vi "HW_Poll_Tracker.vi"(0 "VISA resource name in":refnum<visa-resource-name>="ASRL3::INSTR", 11 "error in":errorcluster) -> (1 "Binary mode status":string, 2 "Coordinate mode status":string, 3 "Matrix mode status":string, 4 "VISA resource name out":refnum<visa-resource-name>, 10 "Read buffer":string, 12 "Sensors response":string, 13 "FPS status":i32, 14 "Port data status":i32, 15 "error out":errorcluster)   [LabVIEW 2016]
panel:
  out "Port data status index":i32
  out "Poll records":u32
  out "FPS target index":i32
  out "Matrix mode index":i32
  out "Coordinate mode index":i32
  out "Binary mode index":i32
  out "Array of tokens":string[](array[string])
  out "token index":i32
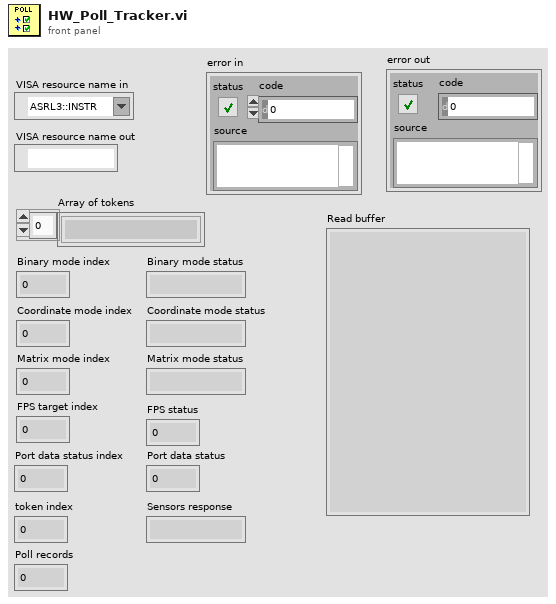
[diagram p1: front panel]
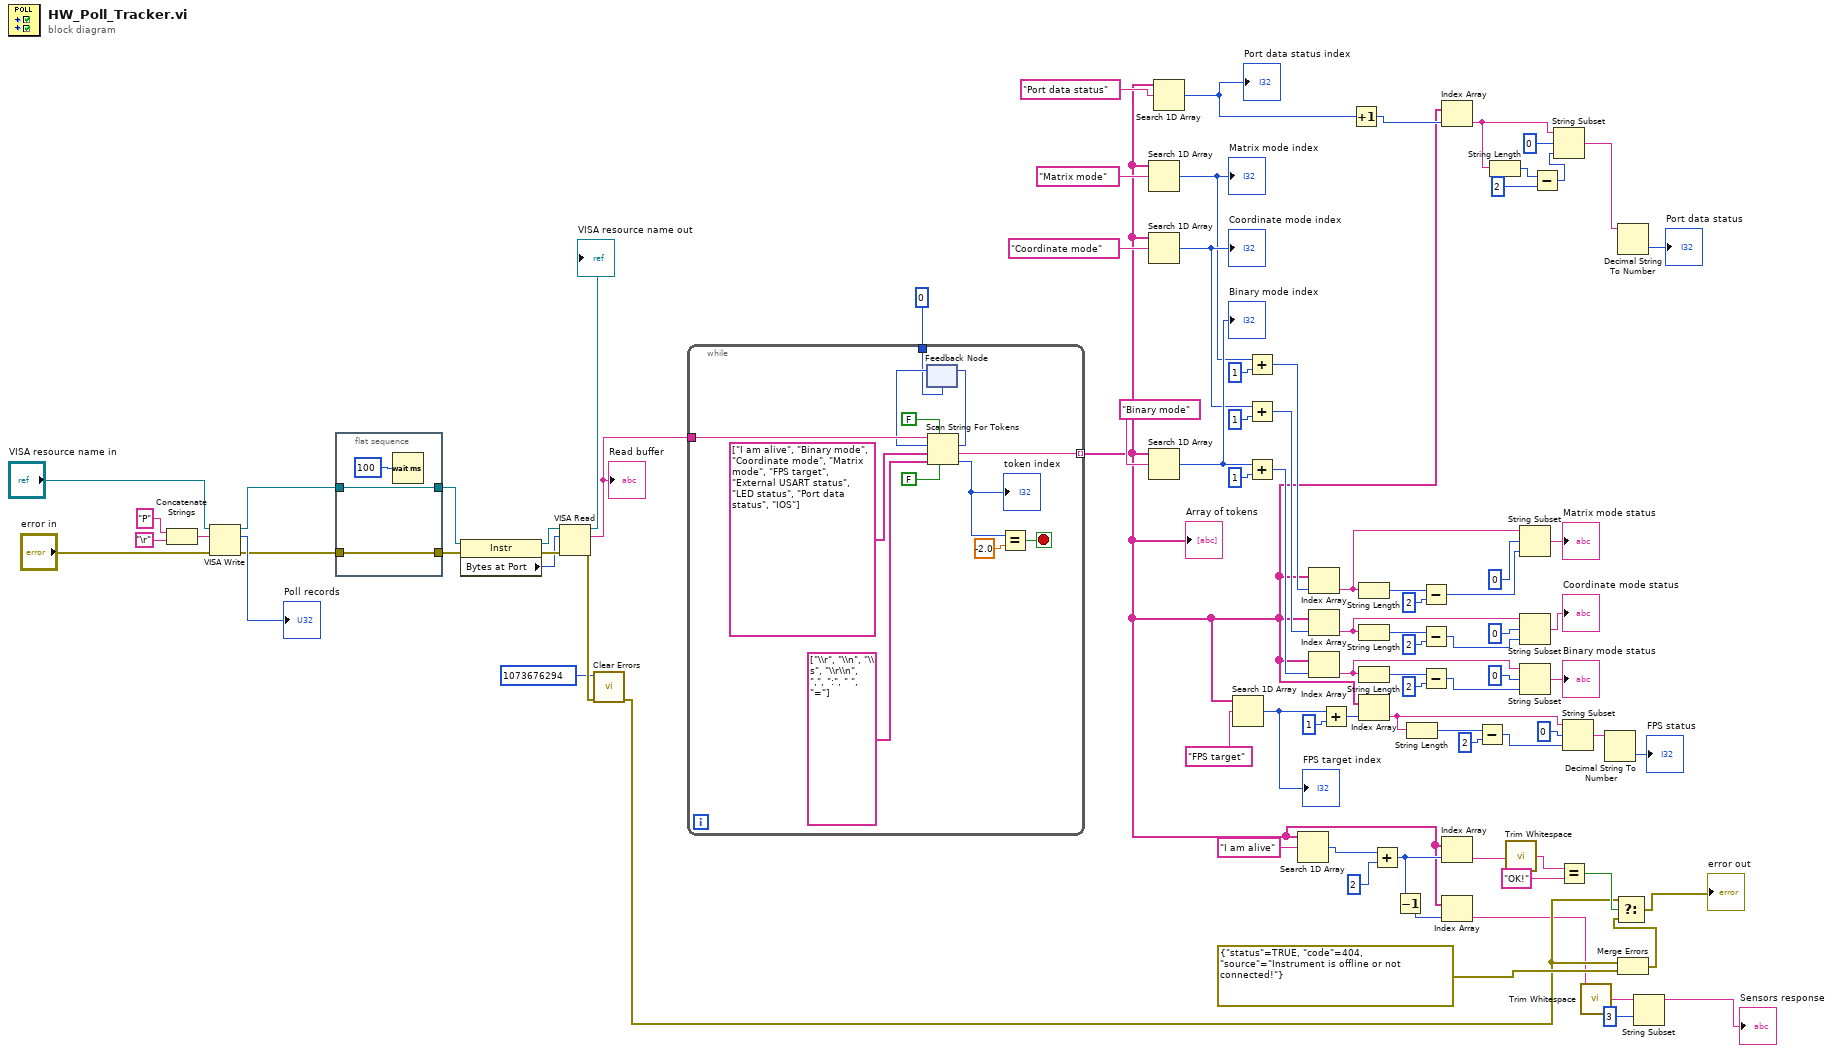
[diagram p0: block diagram]
diagram:
  n1 = Concatenate Strings("P" ("write buffer"), "\r") -> (w85:string)
  n2 = VISA Write(VISA resource name="VISA resource name in", write buffer=w85, error in (no error)="error in") -> (VISA resource name out=w60:refnum<visa-resource-name>, return count=→"Poll records":u32, error out=w58:errorcluster)
  n3 = flat-sequence {
    tunnel: [w89] -> w61
    tunnel: w60 -> [w89]
    tunnel: [w88] -> w59
    tunnel: w58 -> [w88]
    frame #0 {
      n4 = Wait (ms)(milliseconds to wait=u32 100) -> ()  [unwired: 1 out]
    }
  }
  n5 = property class="Instr"(reference=w61, error in=w59) -> (reference out=w83:refnum<visa-resource-name>, error out=w82:errorcluster, "Bytes at Port"=w81:u32)
  n6 = VISA Read(VISA resource name=w83, byte count=w81, error in (no error)=w82) -> (VISA resource name out=→"VISA resource name out":refnum<visa-resource-name>, read buffer=w80:string, error out=w11:errorcluster)  [unwired: 1 out]
  "Read buffer" <- w80
  n7 = call <vilib>:"Clear Errors.vi"("error in (no error)"=w11, "specific error code to clear (0: all)"=1073676294) -> ("error out"=w10:errorcluster)  [unwired: 4 in, 1 out]
  n8 = while {
    tunnel: w80 -> [w102]
    tunnel: [w92] -> w7 mode=indexing
    tunnel: 0 ("offset past token") -> [w91]
    stop <- w98 stop-if-true
    n9 = feedback #1(w91) -> (w99:i32)
    n10 = Scan String For Tokens(4:FALSE ("use cached delim/oper data? (F)"), 5:FALSE ("allow empty tokens? (F)"), 6:string[] ["\\r", "\\n", "\\s", "\\r\\n", ",", ":", " ", "="] ("delimiters"), 7:string[] ["I am alive", "Binary mode", "Coordinate mode", "Matrix mode", "FPS target", "External USART status", "LED status", "Port data status", "IOS"] ("Tokens"), 8:w99, 9:w102) -> (0:w96:i32, 1:w92:string, 2:w100:i32)  [unwired: 1 out]
    "token index" <- w96
    n11 = feedback-in #1(w100) -> ()
    n12 = Equal?(x=w96, y=-2.0) -> (x = y?=w98:bool)
  }
  "Array of tokens" <- w7
  n13 = Search 1D Array(1D array=w7, element="Matrix mode") -> (index of element=w69:i32)  [unwired: 1 in]
  "Matrix mode index" <- w69
  n14 = Search 1D Array(1D array=w7, element="Coordinate mode") -> (index of element=w73:i32)  [unwired: 1 in]
  "Coordinate mode index" <- w73
  n15 = Search 1D Array(1D array=w7, element="Binary mode") -> (index of element=w77:i32)  [unwired: 1 in]
  "Binary mode index" <- w77
  n16 = Search 1D Array(1D array=w7, element="Port data status") -> (index of element=w30:i32)  [unwired: 1 in]
  "Port data status index" <- w30
  n17 = Search 1D Array(1D array=w7, element="FPS target") -> (index of element=w65:i32)  [unwired: 1 in]
  "FPS target index" <- w65
  n18 = Add(x=w69, y=1) -> (x+y=w70:i32)
  n19 = Add(x=w73, y=1) -> (x+y=w74:i32)
  n20 = Add(x=w77, y=1) -> (x+y=w78:i32)
  n21 = Search 1D Array(1D array=w7, element="I am alive") -> (index of element=w20:i32)  [unwired: 1 in]
  n22 = Index Array(array=w7, index=w70) -> (element=w34:string)
  n23 = Index Array(array=w7, index=w74) -> (element=w32:string)
  n24 = Index Array(array=w7, index=w78) -> (element=w54:string)
  n25 = Add(x=w65, y=1) -> (x+y=w66:i32)
  n26 = Increment(x=w30) -> (x+1=w29:i32)
  n27 = String Length(string=w34) -> (length=w49:i32)
  n28 = String Length(string=w32) -> (length=w38:i32)
  n29 = String Length(string=w54) -> (length=w53:i32)
  n30 = Index Array(array=w7, index=w66) -> (element=w33:string)
  n31 = Add(x=w20, y=2) -> (x+y=w8:i32)
  n32 = Decrement(x=w8) -> (x-1=w6:i32)
  n33 = String Length(string=w33) -> (length=w44:i32)
  n34 = Subtract(x=w49, y=2) -> (x-y=w47:i32)
  n35 = Subtract(x=w38, y=2) -> (x-y=w36:i32)
  n36 = Subtract(x=w53, y=2) -> (x-y=w51:i32)
  n37 = Index Array(array=w7, index=w29) -> (element=w28:string)
  n38 = Index Array(array=w7, index=w8) -> (element=w18:string)
  n39 = Index Array(array=w7, index=w6) -> (element=w5:string)
  n40 = Subtract(x=w44, y=2) -> (x-y=w42:i32)
  n41 = String Length(string=w28) -> (length=w27:i32)
  n42 = call <vilib>:"Trim Whitespace.vi"("string"=w18) -> ("trimmed string"=w17:string)  [unwired: 1 in]
  n43 = String Subset(string=w34, offset (0)=0, length (rest)=w47) -> (substring=→"Matrix mode status":string)
  n44 = String Subset(string=w32, offset (0)=0, length (rest)=w36) -> (substring=→"Coordinate mode status":string)
  n45 = String Subset(string=w54, offset (0)=0, length (rest)=w51) -> (substring=→"Binary mode status":string)
  n46 = Subtract(x=w27, y=2) -> (x-y=w25:i32)
  n47 = String Subset(string=w28, offset (0)=0, length (rest)=w25) -> (substring=w23:string)
  n48 = Equal?(x=w17, y="OK!") -> (x = y?=w15:bool)
  n49 = String Subset(string=w33, offset (0)=0, length (rest)=w42) -> (substring=w41:string)
  n50 = call <vilib>:"Trim Whitespace.vi"("string"=w5) -> ("trimmed string"=w4:string)  [unwired: 1 in]
  n51 = Decimal String To Number(string=w41) -> (number=→"FPS status":i32)  [unwired: 2 in, 1 out]
  n52 = Decimal String To Number(string=w23) -> (number=→"Port data status":i32)  [unwired: 2 in, 1 out]
  n53 = Merge Errors(w10, errorcluster {"status"=TRUE, "code"=404, "source"="Instrument is offline or not connected!"} ("error in")) -> (w13:errorcluster)
  n54 = Select(t=w10, s=w15, f=w13) -> (s? t:f=→"error out":errorcluster)
  n55 = String Subset(string=w4, offset (0)=3) -> (substring=→"Sensors response":string)  [unwired: 1 in]
